vi "SV Gen Configure Range and Terminal Settings.vi"(0 "DAQmx Task In":refnum<k21>, 5 "Range and Terminal Settings":T1={"Min Voltage (V)"=-10.0, "Max Voltage (V)"=10.0} {"Max Voltage (V)" format="%#.2p"; "Min Voltage (V)" format="%#.2p"}, 11 "error in (no error)":errorcluster) -> (4 "DAQmx Task Out":refnum<k21>, 15 "error out":errorcluster)   [LabVIEW 2021, in "DAQ_Signal Voltage Generation.lvlib"]
doc: "<B>Configure Range and Terminal Settings </B>\n<B>Range and Temrinal Settings </B>configures the range and terminal settings for all analog output voltage channels where the waveforms are generated for the given DAQmx task. By default all the Analog output channels configuration are kept in \"RSE\" mode."
uses:
  DAQ_Signal Voltage Generation.lvlib
  <resource>/objmgr/daqmx.rc
  Typedefs/Range and Terminal Settings.ctl
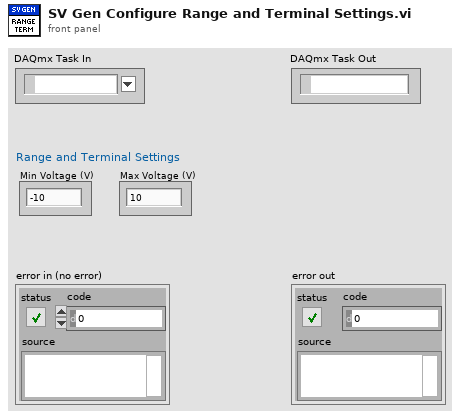
[diagram p1: front panel]
types:
  T1 = typedef "DAQ_Signal Voltage Generation.lvlib/Range and Terminal Settings.ctl" = cluster{"Min Voltage (V)":dbl, "Max Voltage (V)":dbl}
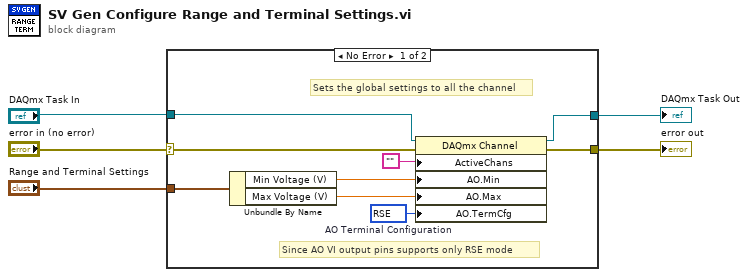
[diagram p0: block diagram]
diagram:
  n1 = case shown="No Error" "error in (no error)" {
    selector: "error in (no error)" -> [w8 w16]
    tunnel: "DAQmx Task In" -> [w10 w15]
    tunnel: "Range and Terminal Settings" -> [w7 _]
    tunnel: [w11 w15] -> w2
    tunnel: [w9 w16] -> w1
    frame No Error {
      w6 = 10083 items=["RSE"=10083, "Differential"=10106, "Pseudodifferential"=12529]  # AO Terminal Configuration
      # "Since AO VI output pins supports only RSE mode"
      # "Sets the global settings to all the channel"
      n2 = Unbundle By Name(w7) -> ("Min Voltage (V)"=w13:dbl, "Max Voltage (V)"=w14:dbl)
      n3 = property class="DAQmx Channel"(reference=w10, error in=w8, "ActiveChans"="", "AO.Min"=w13, "AO.Max"=w14, "AO.TermCfg"=w6) -> (reference out=w11:refnum<k21>, error out=w9:errorcluster)
    }
    frame Error {
      # "Error case - Do Nothing"
    }
  }
  "DAQmx Task Out" <- w2
  "error out" <- w1
